vi "Play+wav+file.vi"() -> ()   [LabVIEW 2011]
uses:
  <vilib>/sound2/lvsound2.llb/Sound File Read Open.vi
  <vilib>/sound2/lvsound2.llb/Sound File Read (DBL).vi
panel:
  in  "Path":path
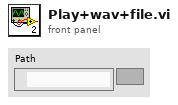
[diagram p1: front panel]
types:
  T1 = typedef "Sound File Refnum.ctl" = refnum<file>
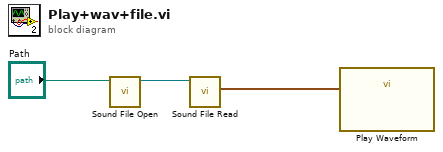
[diagram p0: block diagram]
diagram:
  n1 = call-poly <vilib>:"Sound File Open.vi"("path"="Path") -> ("sound file refnum"=w2:T1)  [unwired: 9 in, 1 out]
  n2 = call-poly <vilib>:"Sound File Read.vi"("sound file refnum"=w2) -> ("data"=w1:waveform(dbl)[])  [unwired: 6 in, 4 out]
  n3 = call "Play Waveform"("Data"=w1) -> ()  [unwired: 18 in, 1 out]
